vi "HovaCAL_Interface_GetComponentConcentration.vi"(8 "error in (no error)":errorcluster caption="Fehler (Eingang, kein Fehler)", 10 "AutoLin MFV Index":u32) -> (0 "error out":errorcluster caption="Fehler (Ausgang)", 2 "AutoLin MFV Index out":u32, 3 "Konzentration":dbl)   [LabVIEW 2020, in "Linearisierung v2.lvlib" / "Gasteiler.lvlib" / "HovaCAL_Interface.lvlib" / "Kommunikation.lvlib"]
uses:
  Kommunikation.lvlib
  Aktion_FGV_HovaCAL_Interface_GetData.ctl
  Aktion_FGV_HovaCAL_Interface_SetData.ctl
  Controls/Pump Concentration Mode.ctl
  Controls/Controls.lvlib
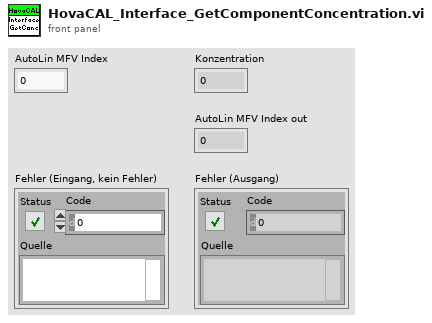
[diagram p1: front panel]
types:
  T1 = typedef "Linearisierung v2.lvlib/Gasteiler.lvlib/HovaCAL_Interface.lvlib/Kommunikation.lvlib/Aktion_FGV_HovaCAL_Interface_GetData.ctl" = enum16{"lesen", "SystemInfo", "MFC Info", "actual Values", "Limits", "first contact"}
  T2 = typedef "Linearisierung v2.lvlib/Gasteiler.lvlib/HovaCAL_Interface.lvlib/Controls.lvlib/Info Cluster.ctl" = cluster{"device":string, "version":string, "number of mfc":i32, "number of pumps":i32, "number of temp controllers":i32, "number of mfs":i32, "number of balances":i32}
  T3 = typedef "Linearisierung v2.lvlib/Gasteiler.lvlib/HovaCAL_Interface.lvlib/Kommunikation.lvlib/Aktion_FGV_HovaCAL_Interface_SetData.ctl" = enum16{"lesen", "Konzentrationen", "Pumpen Parameter", "Pumpe Konzentration", "Pumpe run", "Temperaturen", "Fluss", "Limits", "init"}
  T4 = cluster{"input concentration setpoint":dbl, "output concentration setpoint":dbl}[]
  T5 = cluster{"input concentration setpoint":dbl, "output concentration setpoint":dbl}
  T6 = typedef "Linearisierung v2.lvlib/Gasteiler.lvlib/HovaCAL_Interface.lvlib/Controls.lvlib/Pump Concentration Mode.ctl" = i32
  T7 = typedef "Linearisierung v2.lvlib/Gasteiler.lvlib/HovaCAL_Interface.lvlib/Controls.lvlib/Reagent.ctl" = i32
  T8 = cluster{"concentratio mode":T6, "Reagent":T7, "Molarity":dbl, "density":dbl, "syringe":dbl, "pump_a":dbl}[]
  T9 = typedef "Linearisierung v2.lvlib/Gasteiler.lvlib/HovaCAL_Interface.lvlib/Controls.lvlib/Pump Concentration.ctl" = cluster{"reagent conc SP":dbl, "water conc SP":dbl}
  T10 = cluster{"concentratio mode":T6, "Reagent":T7, "Molarity":dbl, "density":dbl, "syringe":dbl, "pump_a":dbl}
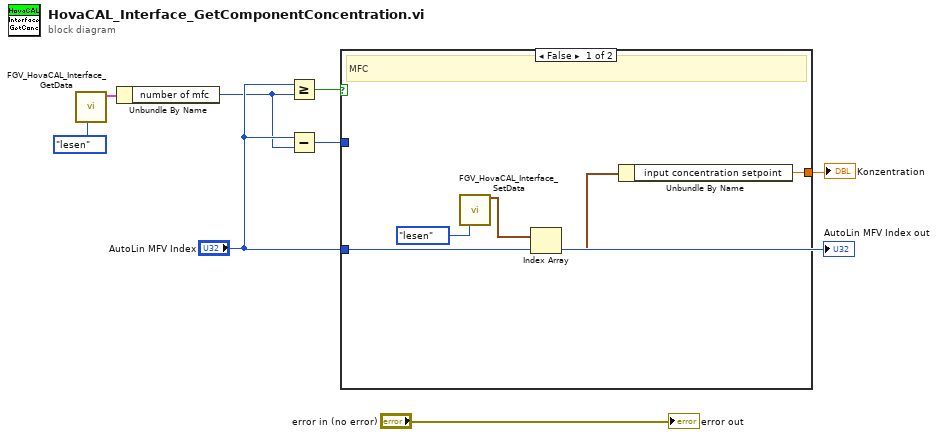
[diagram p0: block diagram]
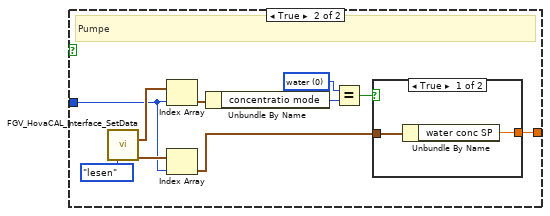
[diagram p2: hidden frame]
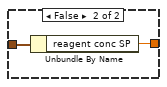
[diagram p3: hidden frame]
diagram:
  n1 = call "FGV_HovaCAL_Interface_GetData.vi"("Aktion"=Aktion_FGV_HovaCAL_Interface_GetData."lesen") -> ("System Cluster out"=w7:T2)  [unwired: 6 in, 4 out]
  n2 = Unbundle By Name(w7) -> ("number of mfc"=w5:i32)
  n3 = Greater Or Equal?(x="AutoLin MFV Index", y=w5) -> (x >= y?=w4:bool)
  n4 = Subtract(x="AutoLin MFV Index", y=w5) -> (x-y=w3:u32)
  n5 = case shown="False" w4 {
    tunnel: "AutoLin MFV Index" -> [w13 _]
    tunnel: w3 -> [_ w15]
    tunnel: [w9 w20] -> w1
    frame False {
      # "MFC"
      n6 = call "FGV_HovaCAL_Interface_SetData.vi"("Aktion"=Aktion_FGV_HovaCAL_Interface_SetData."lesen") -> ("Set Values Cluster out"=w10:T4)  [unwired: 8 in, 6 out]
      n7 = Index Array(array=w10, index=w13) -> (element=w11:T5)
      n8 = Unbundle By Name(w11) -> ("input concentration setpoint"=w9:dbl)
    }
    frame True {
      w17 = T6 0 items=["water", "reagent"] ("x")
      # "Pumpe"
      n9 = call "FGV_HovaCAL_Interface_SetData.vi"("Aktion"=Aktion_FGV_HovaCAL_Interface_SetData."lesen") -> ("PumpMode-Cluster out"=w16:T8, "Pump Concentrations-Cluster out"=w21:T9[])  [unwired: 8 in, 5 out]
      n10 = Index Array(array=w16, index=w15) -> (element=w19:T10)
      n11 = Index Array(array=w21, index=w15) -> (element=w22:T9)
      n12 = Unbundle By Name(w19) -> ("concentratio mode"=w18:T6)
      n13 = Equal?(x=w17, y=w18) -> (x = y?=w14:bool)
      n14 = case shown="True" w14 {
        tunnel: w22 -> [w25 w27]
        tunnel: [w24 w26] -> w20
        frame True {
          n15 = Unbundle By Name(w25) -> ("water conc SP"=w24:dbl)
        }
        frame False {
          n16 = Unbundle By Name(w27) -> ("reagent conc SP"=w26:dbl)
        }
      }
    }
  }
  "Konzentration" <- w1
  "error out" <- "error in (no error)"
  "AutoLin MFV Index out" <- "AutoLin MFV Index"
